vi "Initialize.vi"(7 "Fallback File Path":path, 8 "error in (no error)":errorcluster, 9 "Dataset RID":string, 10 "Token":string) -> (0 "error out":errorcluster, 3 "Nominal Streaming out":refnum<class "Stream.lvclass">)   [LabVIEW 2020, in "Nominal Streaming.lvlib" / "Stream.lvclass"]
uses:
  Stream.lvclass
  Stream.lvclass/Stream.ctl
  bin/lib_nominal-streaming-lv_64.dll
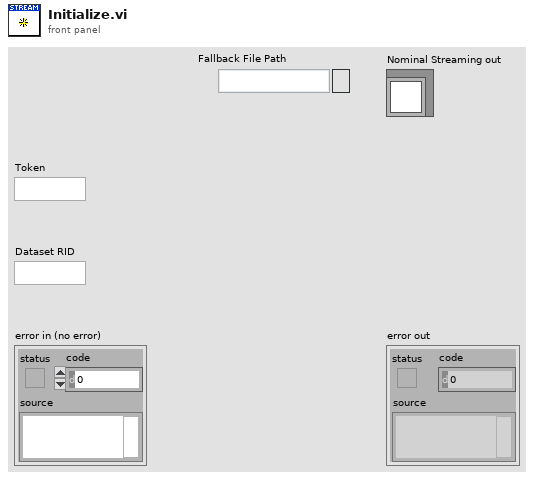
[diagram p1: front panel]
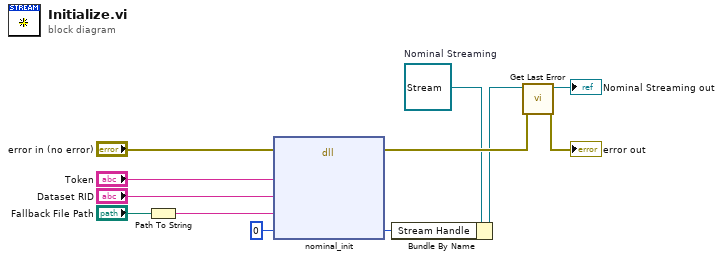
[diagram p0: block diagram]
diagram:
  w1 = refnum<class "Stream.lvclass"> refnum  # Nominal Streaming
  n1 = Path To String(path="Fallback File Path") -> (string=w11:string)
  n2 = dll-call lib="C:/code/nominal-streaming-labview-ffi/lv_src/bin/lib_nominal-streaming-lv_*.*" fn="nominal_init"(error in="error in (no error)", "token"="Token", "dataset_rid"="Dataset RID", "fallback_file_path"=w11, "out_stream_handle"=u64 0) -> (error out=w5:errorcluster, "out_stream_handle"=w6:u64)  [unwired: 6 in, 1 out]
  n3 = Bundle By Name(cluster=w1, "Stream Handle"=w6) -> (w3:refnum<class "Stream.lvclass">)
  n4 = call "Get Last Error.vi"("error in (no error)"=w5, "Nominal Streaming in"=w3) -> ("error out"=→"error out":errorcluster, "Nominal Streaming out"=→"Nominal Streaming out":refnum<class "Stream.lvclass">)  [unwired: 8 in]
